vi "Tektronix Series Read Horizontal Settings.vi"() -> ()   [LabVIEW 2021]
doc: "This example VI illustrates how to configure and query horizontal properties."
uses:
  <instrlib>/Tektronix MSO5X Series/Tektronix MSO5X Series.lvlib
panel:
  out "SMU Scope Interpolation Ratio":dbl
  out "SMU Scope Timebase Duration (s)":dbl
  out "SMU Scope Division Number":i32
  in  "SMU Scope":refnum<visa-resource-name>
  in  "error in":errorcluster
  out "error out":errorcluster
  in  "Maximum Record Length":dbl=250000000.0 format="%#_6e"
  in  "Sample Rate":dbl=3125000000.0
  in  "Control Type":i32(ring) items=["Horizontal Scale", "Record Length"]
  out "Load Division Number":i32
  out "Load Timebase Duration (s)":dbl
  out "Load Interpolation Ratio":dbl
  in  "Load Scope":refnum<visa-resource-name>
  # "(c) 2023  National Instruments Corporation.  ALL RIGHTS RESERVED."
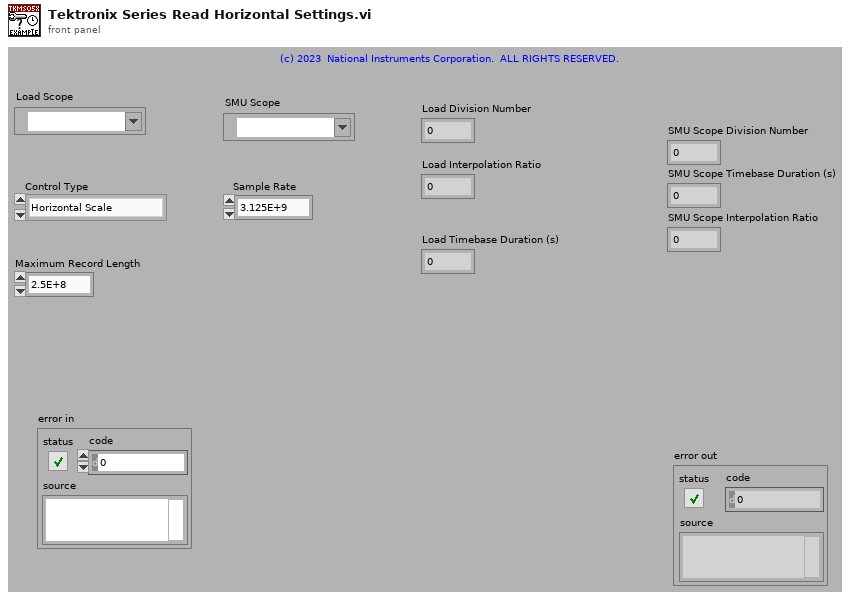
[diagram p1: front panel]
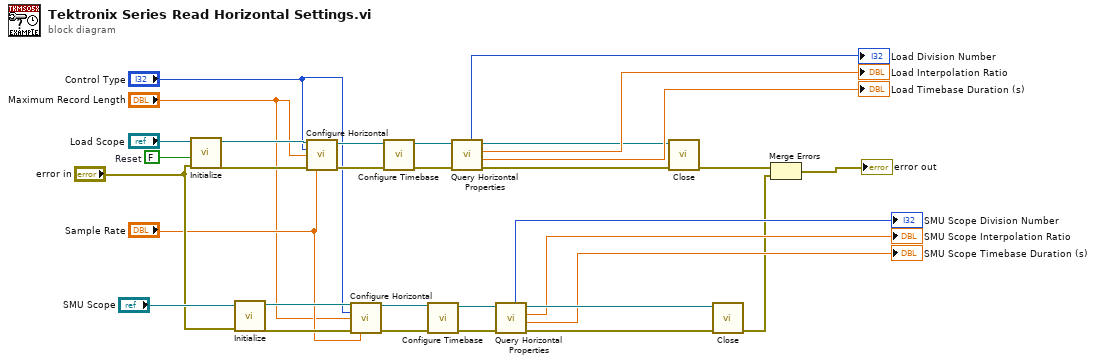
[diagram p0: block diagram]
diagram:
  w31 = FALSE  # Reset
  n1 = call <instrlib>:"Initialize.vi"("error in (no error)"="error in", "Reset (True)"=w31, "VISA resource name"="Load Scope") -> ("error out"=w29:errorcluster, "VISA resource name out"=w30:refnum<visa-resource-name>)  [unwired: 7 in]
  n2 = call <instrlib>:"Initialize.vi"("error in (no error)"="error in", "VISA resource name"="SMU Scope") -> ("error out"=w15:errorcluster, "VISA resource name out"=w10:refnum<visa-resource-name>)  [unwired: 8 in]
  n3 = call <instrlib>:"Configure Horizontal.vi"("VISA resource name"=w30, "Control Type (0: Horizontal Scale)"="Control Type", "Maximum Record Length (2.5E+8)"="Maximum Record Length", "error in (no error)"=w29, "Sample Rate (3.125E+9)"="Sample Rate") -> ("VISA resource name out"=w23:refnum<visa-resource-name>, "error out"=w22:errorcluster)  [unwired: 9 in]
  n4 = call <instrlib>:"Configure Horizontal.vi"("VISA resource name"=w10, "Control Type (0: Horizontal Scale)"="Control Type", "Maximum Record Length (2.5E+8)"="Maximum Record Length", "error in (no error)"=w15, "Sample Rate (3.125E+9)"="Sample Rate") -> ("VISA resource name out"=w11:refnum<visa-resource-name>, "error out"=w17:errorcluster)  [unwired: 9 in]
  n5 = call <instrlib>:"Configure Timebase.vi"("error in (no error)"=w22, "VISA resource name"=w23) -> ("error out"=w21:errorcluster, "VISA resource name out"=w20:refnum<visa-resource-name>)  [unwired: 8 in]
  n6 = call <instrlib>:"Configure Timebase.vi"("error in (no error)"=w17, "VISA resource name"=w11) -> ("error out"=w18:errorcluster, "VISA resource name out"=w12:refnum<visa-resource-name>)  [unwired: 8 in]
  n7 = call <instrlib>:"Query Horizontal Properties.vi"("error in (no error)"=w21, "VISA resource name"=w20) -> ("error out"=w24:errorcluster, "Timebase Duration (s)"=→"Load Timebase Duration (s)":dbl, "Interpolation Ratio"=→"Load Interpolation Ratio":dbl, "VISA resource name out"=w25:refnum<visa-resource-name>, "Division Number"=→"Load Division Number":i32)  [unwired: 5 in]
  n8 = call <instrlib>:"Query Horizontal Properties.vi"("error in (no error)"=w18, "VISA resource name"=w12) -> ("error out"=w16:errorcluster, "Timebase Duration (s)"=→"SMU Scope Timebase Duration (s)":dbl, "Interpolation Ratio"=→"SMU Scope Interpolation Ratio":dbl, "VISA resource name out"=w13:refnum<visa-resource-name>, "Division Number"=→"SMU Scope Division Number":i32)  [unwired: 5 in]
  n9 = call <instrlib>:"Close.vi"("error in (no error)"=w24, "VISA resource name"=w25) -> ("error out"=w19:errorcluster)  [unwired: 9 in]
  n10 = call <instrlib>:"Close.vi"("error in (no error)"=w16, "VISA resource name"=w13) -> ("error out"=w1:errorcluster)  [unwired: 9 in]
  n11 = Merge Errors(w19, w1) -> (→"error out":errorcluster)
